vi "setParameters.vi"(10 "Parameters":T1, 11 "EnableCommand in":refnum<class "EnableCommand.lvclass">) -> (3 "EnableCommand out":refnum<class "EnableCommand.lvclass">)   [LabVIEW 2016, in "EnableCommand.lvclass"]
uses:
  EnableCommand.lvclass
  Communicator/Topics/CommandEnable.ctl
  Communicator/Topics/CommandId.ctl
  EnableCommand.lvclass/EnableCommand.ctl
  Communicator/M1M3Communicator.lvlib
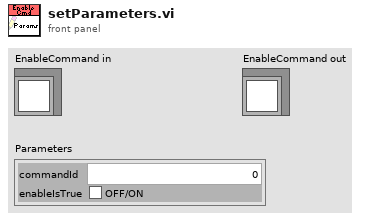
[diagram p1: front panel]
types:
  T1 = typedef "M1M3Communicator.lvlib/CommandEnable.ctl" = cluster{"commandId":T2, "enableIsTrue":bool}
  T2 = typedef "M1M3Communicator.lvlib/CommandId.ctl" = i32
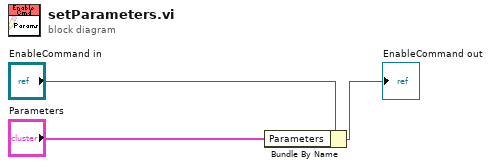
[diagram p0: block diagram]
diagram:
  n1 = Bundle By Name(cluster="EnableCommand in", "Parameters"="Parameters") -> (→"EnableCommand out":refnum<class "EnableCommand.lvclass">)
